vi "Get State.vi"(6 "Controller name":string, 8 "error in (no error)":errorcluster, 11 "Combined Measurement in":refnum<class "Combined Measurement.lvclass">) -> (0 "error out":errorcluster, 1 "Result ready":bool, 2 "Armed":bool, 3 "Combined Measurement out":refnum<class "Combined Measurement.lvclass">, 4 "Check again":bool)   [LabVIEW 2021, in "Combined Measurement.lvclass"]
uses:
  Combined Measurement.lvclass
  Measurements/Response Synchronizer/Response Synchronizer.lvclass
  Combined Measurement.lvclass/Combined Measurement.ctl
  Continuous Recorder Actor/Continuous Recorder Actor.lvclass
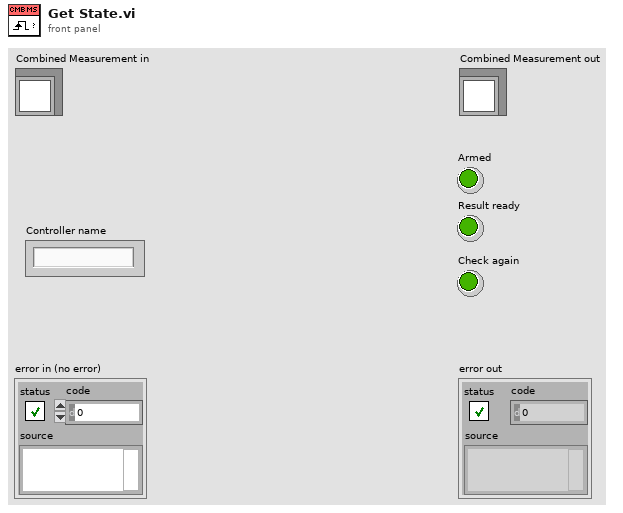
[diagram p1: front panel]
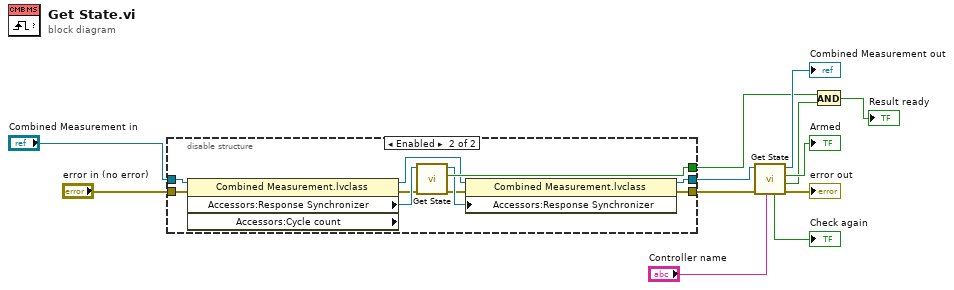
[diagram p0: block diagram]
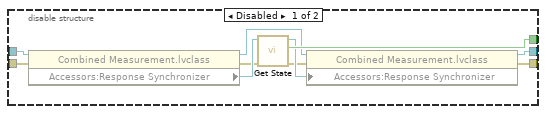
[diagram p2: hidden frame]
diagram:
  n1 = disable-structure shown="Enabled" {
    disable-tunnel: "error in (no error)" -> [w22 w32]
    disable-tunnel: "Combined Measurement in" -> [w21 w31]
    disable-tunnel: [w18 w28] -> w5
    disable-tunnel: [w14 w23] -> w6
    disable-tunnel: [w13 w24] -> w1
    frame Disabled {
      n2 = property class="Combined Measurement.lvclass"(reference=w21, error in=w22) -> (reference out=w15:refnum<class "Combined Measurement.lvclass">, error out=w19:errorcluster, "Accessors:Response Synchronizer"=w20:refnum<class "Response Synchronizer.lvclass">)
      n3 = call-dynamic "Get State.vi"("error in (no error)"=w19, "Response Synchronizer in"=w20) -> ("error out"=w16:errorcluster, "Result ready"=w18:bool, "Response Synchronizer out"=w17:refnum<class "Response Synchronizer.lvclass">)  [unwired: 4 in, 3 out]
      n4 = property class="Combined Measurement.lvclass"(reference=w15, error in=w16, "Accessors:Response Synchronizer"=w17) -> (reference out=w14:refnum<class "Combined Measurement.lvclass">, error out=w13:errorcluster)
    }
    frame Enabled {
      n5 = property class="Combined Measurement.lvclass" props=["Accessors:Response Synchronizer", "Accessors:Cycle count"](reference=w31, error in=w32) -> (reference out=w27:refnum<class "Combined Measurement.lvclass">, error out=w29:errorcluster, "Accessors:Response Synchronizer"=w30:refnum<class "Response Synchronizer.lvclass">)  [unwired: 1 out]
      n6 = call-dynamic "Get State.vi"("error in (no error)"=w29, "Response Synchronizer in"=w30) -> ("error out"=w25:errorcluster, "Result ready"=w28:bool, "Response Synchronizer out"=w26:refnum<class "Response Synchronizer.lvclass">)  [unwired: 4 in, 3 out]
      n7 = property class="Combined Measurement.lvclass"(reference=w27, error in=w25, "Accessors:Response Synchronizer"=w26) -> (reference out=w23:refnum<class "Combined Measurement.lvclass">, error out=w24:errorcluster)
    }
  }
  n8 = call-parent "Get State.vi"("Controller name"="Controller name", "error in (no error)"=w1, "Instrument Actor in"=w6) -> ("error out"=→"error out":errorcluster, "Result ready"=w4:bool, "Armed"=→"Armed":bool, "Instrument Actor out"=→"Combined Measurement out":refnum<class "Combined Measurement.lvclass">, "Check again"=→"Check again":bool)  [unwired: 4 in]
  n9 = And(x=w5, y=w4) -> (x .and. y?=→"Result ready":bool)
